vi "parse error message.vi"(8 "error in":errorcluster, 11 "message data":string) -> (0 "error out":errorcluster, 2 "system error":errorcluster)   [LabVIEW 2013, in "TBD message service.lvlib"]
doc: "Parses error information sent by the Engine Service."
uses:
  TBD message service.lvlib
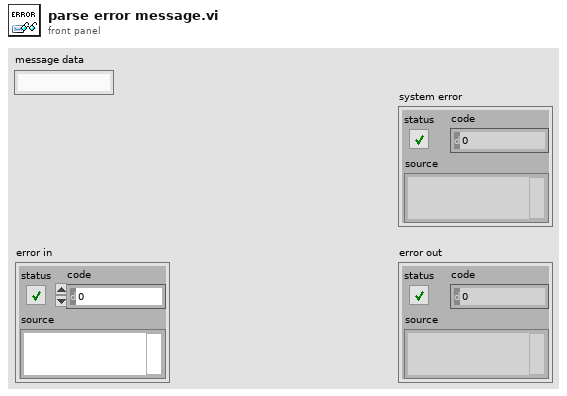
[diagram p1: front panel]
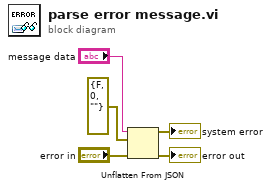
[diagram p0: block diagram]
diagram:
  n1 = Unflatten From JSON(JSON string="message data", type and defaults=errorcluster {"status"=FALSE, "code"=0, "source"=""} ("error constant"), error in (no error)="error in") -> (value=→"system error":errorcluster, error out=→"error out":errorcluster)  [unwired: 4 in]
